vi "find_element.vi"   [LabVIEW 2018]
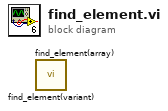
[diagram p0: block diagram]
diagram:
  n1 = call "find_element(variant).vi"() -> ()  [unwired: 8 in, 4 out]
  n2 = call "find_element(array).vi"() -> ()  [unwired: 8 in, 4 out]
